vi "Multi-Device Synch-AI and AO-Multi Rate-Trig Skew Correction.vi"() -> ()   [LabVIEW 2011, in "run.lvlib"]
doc: "I. Description:\nThis example demonstrates how to synchronize an Analog Input Voltage and Analog Output Voltage task using Reference Clock Synchronization and Trigger Skew Correction.\n\nII. Instructions for Running:\n1. Select the Analog Input physical channel to correspond to where your signal is input on the DAQ device. Select the Analog Output physical channel to correspond to where your signal is output on the DAQ device.\n2. Enter the minimum and maximum voltage ranges for both input and output.\nNote: For better accuracy try to match the ranges to the expected voltage levels of the measured and generated signals.\n3. Set the rate of the acquisition of the input task.\nNote: The rate should be at least twice as fast as the maximum frequency component of the signal being acquired.\n4. Set the rate of the generation of the output task.\n5. Set the System Delay of the system being tested. This is the expected delay from the stimulus from the Output task to the measured result on the Input task.\n6. Set the number of Samples to Read per iteration of the while loop.\n7. Set the reference clock source and rate of the system. The defaults are appropriate for PXIe devices.\n8. Configure the signal to generate on the Output task.\n\nIII. Block Diagram Steps:\n1. Create an analog input voltage channel. Also, create an analog output voltage channel.\n2. Set the rate for the sample clock. Additionally, define the sample mode to be continuous. Also, set the sample clock rate for the signal generation.\n3. Synchronize the tasks using Reference Clock Synchronization and Trigger Skew Correction. The defaults for Reference Clock Source and Rate are appropriate for PXIe devices.\n4. Configure the System Delay of the system.\n5. Use the Basic Function Generator VI to create the signal to be generated.\n6. Call the Start VI to arm the two functions. Make sure the analog output is armed before the analog input. This will ensure both will start at the same time.\n7. Read the waveform data in a loop until the user hits the stop button or an error occurs. The Is Task Done? VI is used to check for errors in the Analog Output Task.\n8. Call the Stop VI to Stop the Tasks.\n9. Call the Clear VI to Clear the Tasks.\n10. Use the popup dialog box to display an error if any.\n\nIV. I/O Connections Overview:\nMake sure your signal input and output terminals match the Physical Channel I/O controls. \n\nIf you have a PXIe chassis, ensure it has been properly identified in MAX. If you have devices with a RTSI bus, ensure they are connected with a RTSI cable and that the RTSI cable is registered in MAX."
uses:
  Hal/testing/run.lvlib
  <vilib>/Utility/error.llb/DialogType.ctl
  <vilib>/DAQmx/read.llb/DAQmx Read (Analog 2D DBL NChan NSamp).vi
  <vilib>/DAQmx/create/channels.llb/DAQmx Create Channel (AI-Voltage-Basic).vi
  <vilib>/DAQmx/configure/timing.llb/DAQmx Timing (Sample Clock).vi
  <vilib>/DAQmx/configure/trigger.llb/DAQmx Start Trigger (Digital Edge).vi
  <vilib>/DAQmx/miscellaneous.llb/DAQmx Fill In Error Info.vi
panel:
  in  "Repeat":i32=100
  in  "samples per channel":i32=25000
  in  "Clock Rate":dbl=250000.0 format="%0.2f"
  in  "trigger":tag="/Daq/PFI0"
  in  "file path (dialog if empty)":path=path "C:/Users/chipper/Desktop/data/sideBands.txt"
  out "Measurement":dbl[][](graph)
  in  "Samples to Read":i32=25000
  in  "Maximum Value":dbl=10.0 caption="Input Maximum Value" format="%0.2f"
  in  "Minimum Value":dbl=-10.0 caption="Input Minimum Value" format="%0.2f"
  in  "Physical Channels":tag="Daq/ai1" caption="Input Physical Channel"
  # "For instructions, select Help>>Show Context Help"
  # "Channel Parameters"
  # "Timing Parameters"
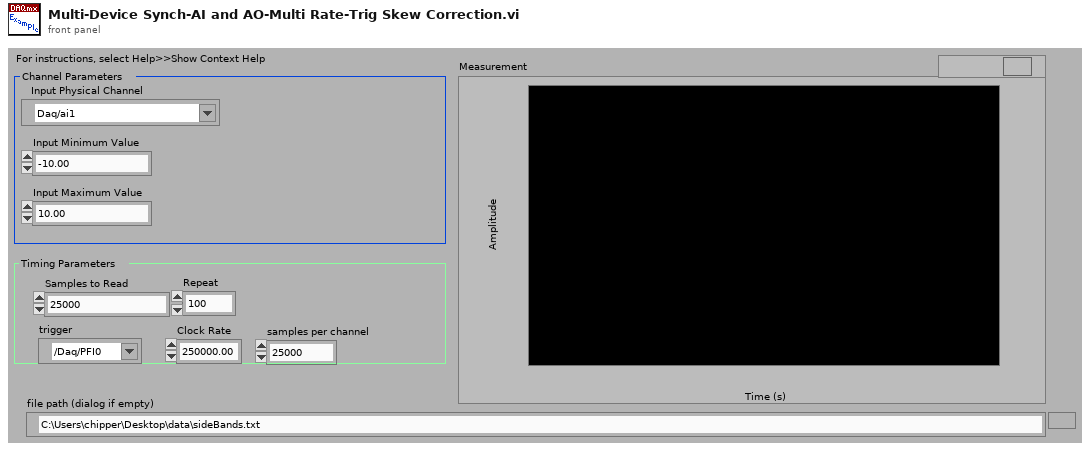
[diagram p1: front panel]
types:
  T1 = typedef "DialogType.ctl" = u16
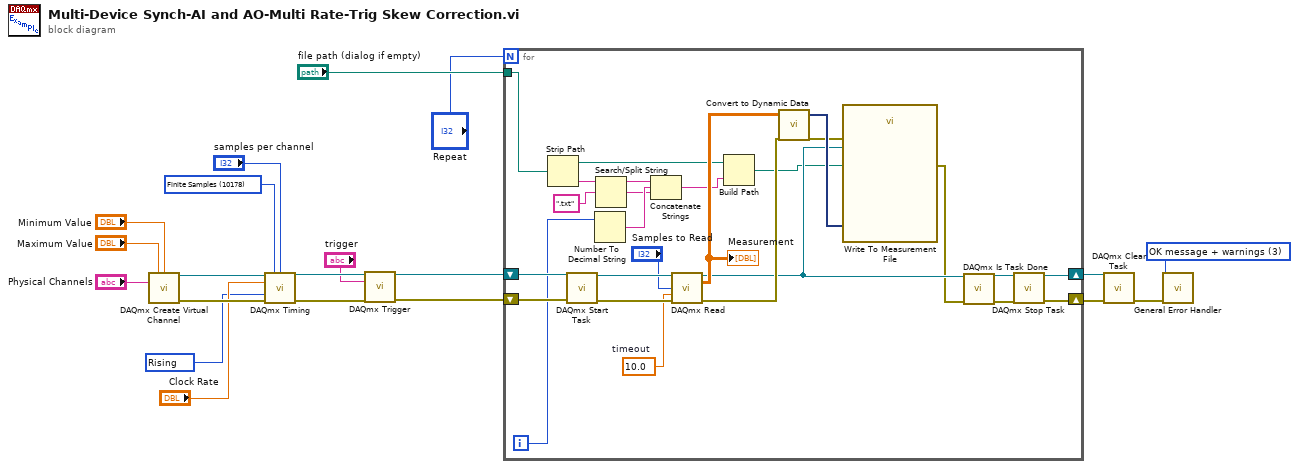
[diagram p0: block diagram]
diagram:
  w7 = 10280 items=["Rising"=10280, "Falling"=10171] ("active edge")
  w15 = T1 3 items=["no dialog", "OK message", "continue or stop message", "OK message + warnings", "continue/stop + warnings"] ("type of dialog (OK msg:1)")
  w18 = 10178 items=["Finite Samples"=10178, "Continuous Samples"=10123] ("sample mode")
  n1 = call-poly <vilib>:"DAQmx Create Virtual Channel.vi"("maximum value"="Maximum Value", "minimum value"="Minimum Value", "physical channels"="Physical Channels") -> ("task out"=w16:refnum<k21>, "error out"=w17:errorcluster)  [unwired: 11 in]
  n2 = call-poly <vilib>:"DAQmx Timing.vi"("task/channels in"=w16, "sample mode"=w18, "samples per channel"="samples per channel", "rate"="Clock Rate", "active edge"=w7, "error in"=w17) -> ("task out"=w11:refnum<k21>, "error out"=w10:errorcluster)  [unwired: 8 in]
  n3 = call-poly <vilib>:"DAQmx Trigger.vi"("task/channels in"=w11, "source"="trigger", "error in"=w10) -> ("task out"=w5:refnum<k21>, "error out"=w4:errorcluster)  [unwired: 11 in]
  n4 = for {
    N: "Repeat" -> [_]
    tunnel: "file path (dialog if empty)" -> [w30]
    shift-right: [w32] -> w2
    shift-left: w5 -> [w43]
    shift-right: [w31] -> w1
    shift-left: w4 -> [w42]
    i -> [w27]
    w41 = 10.0  # timeout
    n5 = Strip Path(path=w30) -> (stripped path=w22:path, name=w29:string)
    n6 = call <vilib>:"DAQmx Start Task.vi"("task/channels in"=w43, "error in"=w42) -> ("task out"=w45:refnum<k21>, "error out"=w44:errorcluster)  [unwired: 12 in]
    n7 = Number To Decimal String(number=w27) -> (decimal integer string=w25:string)  [unwired: 1 in]
    n8 = Search/Split String(string=w29, search string/char (-)=".txt") -> (substring before match=w26:string, match + rest of string=w24:string)  [unwired: 1 in, 1 out]
    n9 = Concatenate Strings(w26, w25, w24) -> (w23:string)
    n10 = call-poly <vilib>:"DAQmx Read.vi"("task/channels in"=w45, "number of samples per channel"="Samples to Read", "timeout"=w41, "error in"=w44) -> ("task out"=w36:refnum<k21>, "data"=w39:dbl[][], "error out"=w37:errorcluster)  [unwired: 9 in]
    "Measurement" <- w39
    n11 = Build Path(base path=w22, name or relative path=w23) -> (appended path=w21:path)
    n12 = call "Convert to Dynamic Data"("2D Array"=w39) -> ("Dynamic Data Type"=w38:dynamicdata)  [unwired: 3 in]
    n13 = call "Write To Measurement File"("Signals"=w38, "error in (no error)"=w37, "Filename"=w21, "DAQmx Task"=w36) -> ("error out"=w35:errorcluster)  [unwired: 13 in, 2 out]
    n14 = call <vilib>:"DAQmx Is Task Done.vi"("task/channels in"=w36, "error in"=w35) -> ("task out"=w34:refnum<k21>, "error out"=w33:errorcluster)  [unwired: 11 in, 1 out]
    n15 = call <vilib>:"DAQmx Stop Task.vi"("task/channels in"=w34, "error in"=w33) -> ("task out"=w32:refnum<k21>, "error out"=w31:errorcluster)  [unwired: 12 in]
  }
  n16 = call <vilib>:"DAQmx Clear Task.vi"("task in"=w2, "error in"=w1) -> ("error out"=w13:errorcluster)  [unwired: 13 in]
  n17 = call <vilib>:"General Error Handler.vi"("type of dialog (OK msg:1)"=w15, "error in (no error)"=w13) -> ()  [unwired: 9 in, 5 out]
